vi "GetDatabase.vi"(8 "error in (no error)":errorcluster, 10 "databaseName":string="hitran", 11 "MongoDB-Client in":refnum<class "MongoDB-Client.lvclass">) -> (0 "error out":errorcluster, 2 "MongoDB-Database":refnum<class "MongoDB-Database.lvclass">, 3 "MongoDB-Client out":refnum<class "MongoDB-Client.lvclass">)   [LabVIEW 2016, in "MongoDB-Client.lvlib" / "MongoDB-Client.lvclass"]
uses:
  MongoDB-Client.lvclass
  D:/Users/blume/Desktop/LV/MongoDB-Driver/MLV DLLs/MongoLabVIEW.dll
  LV/MongoDB-Driver/MLV DLLs/MongoLabVIEW.dll
  MongoDB-Database/MongoDB-Database/MongoDB-Database.lvclass
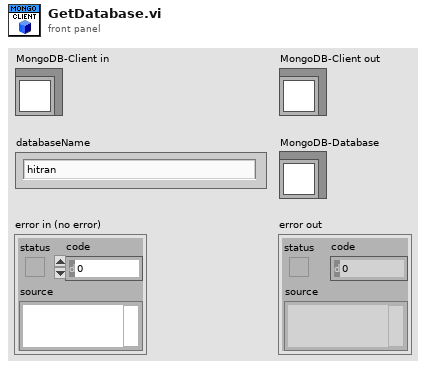
[diagram p1: front panel]
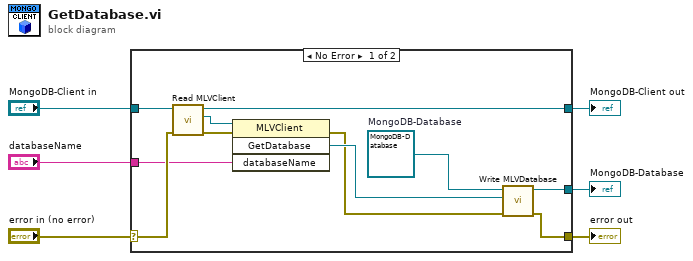
[diagram p0: block diagram]
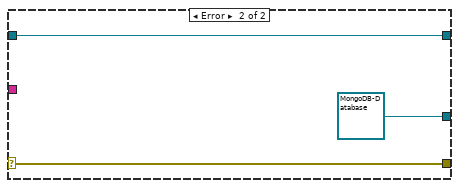
[diagram p2: hidden frame]
diagram:
  n1 = case shown="No Error" "error in (no error)" {
    selector: "error in (no error)" -> [w14 w20]
    tunnel: [w7 w20] -> w5
    tunnel: [w16 w19] -> w3
    tunnel: "MongoDB-Client in" -> [w17 w19]
    tunnel: "databaseName" -> [w12 _]
    tunnel: [w8 refnum<class "MongoDB-Database.lvclass"> refnum ("MongoDB-Database out")] -> w1
    frame No Error {
      w11 = refnum<class "MongoDB-Database.lvclass"> refnum  # MongoDB-Database
      n2 = call "Read MLVClient.vi"("error in (no error)"=w14, "MongoDB-Client in"=w17) -> ("error out"=w13:errorcluster, "MLVClient"=w15:refnum<k24>, "MongoDB-Client out"=w16:refnum<class "MongoDB-Client.lvclass">)  [unwired: 7 in]
      n3 = invoke class="MLVClient" method="GetDatabase"(reference=w15, error in=w13, "databaseName"=w12) -> (error out=w9:errorcluster, "GetDatabase"=w10:refnum<k24>)  [unwired: 1 in, 2 out]
      n4 = call "Write MLVDatabase.vi"("error in (no error)"=w9, "MLVDatabase"=w10, "MongoDB-Database in"=w11) -> ("error out"=w7:errorcluster, "MongoDB-Database out"=w8:refnum<class "MongoDB-Database.lvclass">)  [unwired: 7 in]
    }
    frame Error {
    }
  }
  "error out" <- w5
  "MongoDB-Client out" <- w3
  "MongoDB-Database" <- w1
